vi "Dialog Window with Option.vi"(8 "Error In":errorcluster, 9 "Button 2 (Cancel)":string="Cancel", 10 "Button 1 (OK)":string="OK", 11 "Message":string) -> (0 "Error Out":errorcluster, 1 "Cancelled?":bool, 3 "OK?":bool)   [LabVIEW 2019]
panel:
  in  "Cancel":bool
  in  "OK":bool
  in  "Do not show this warning again":bool
  out "Displayed Message":string
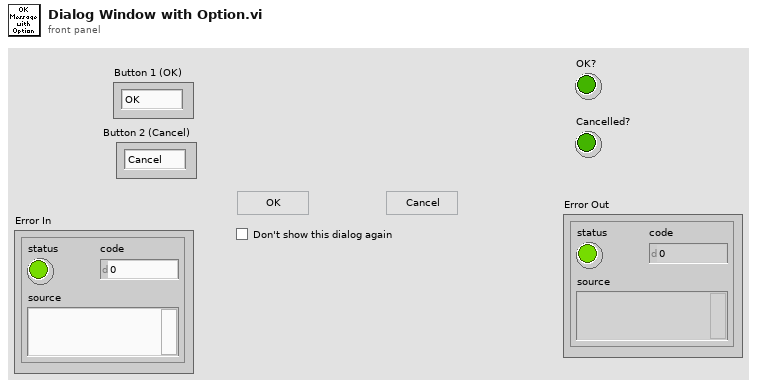
[diagram p1: front panel]
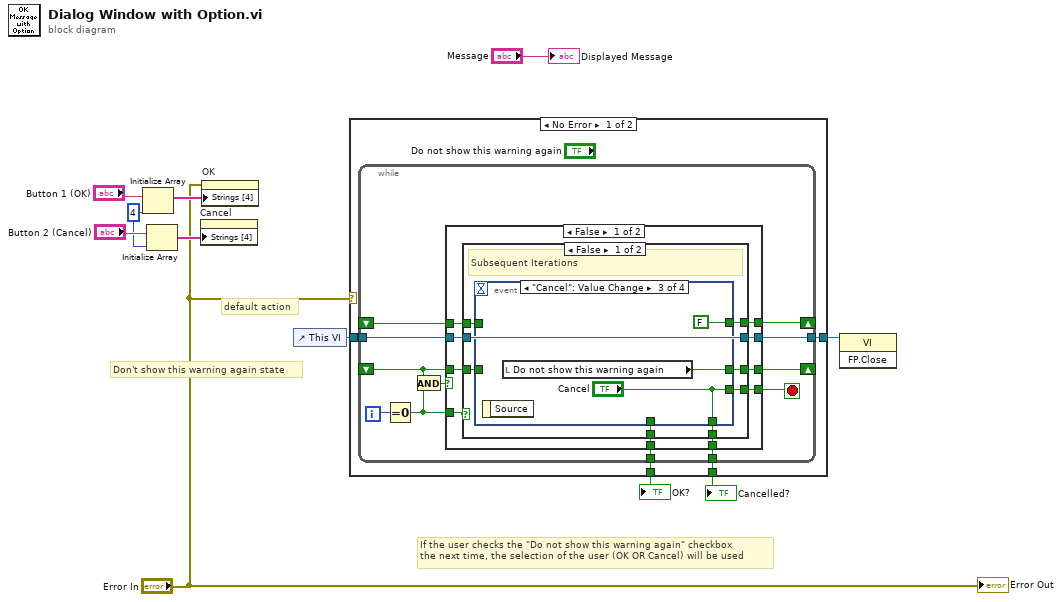
[diagram p0: block diagram]
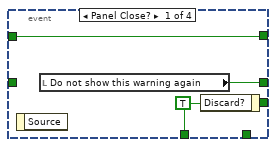
[diagram p2: hidden frame]
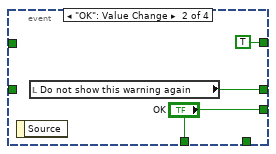
[diagram p3: hidden frame]
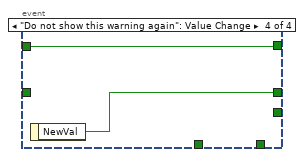
[diagram p4: hidden frame]
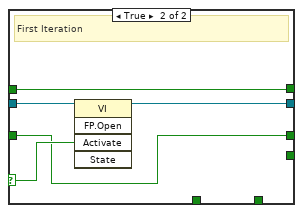
[diagram p5: hidden frame]
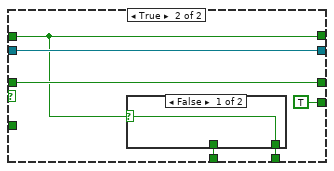
[diagram p6: hidden frame]
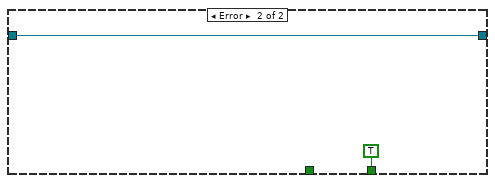
[diagram p8: hidden frame]
diagram:
  w3 = 4 ("dimension size")
  # "default action"
  # "Don't show this warning again state"
  # "If the user checks the \"Do not show this warning again\" checkbox\nthe next time, the selection of the user (OK OR Cancel) will be used"
  n1 = Initialize Array("Button 1 (OK)", w3) -> (w5:string[])
  n2 = Initialize Array("Button 2 (Cancel)", w3) -> (w2:string[])
  n3 = property on="Cancel" class="Bool"("Strings [4]"=w2) -> ()  [unwired: 2 in, 2 out]
  n4 = property on="OK" class="Bool"(error in="Error In", "Strings [4]"=w5) -> ()  [unwired: 1 in, 2 out]
  n5 = control-ref of="This VI"() -> (w10:refnum<vi>)
  n6 = case shown="No Error" "Error In" {
    tunnel: w10 -> [w15 w71]
    tunnel: [w14 w71] -> w9
    tunnel: [w13 _] -> w8
    tunnel: [w12 TRUE ("Cancel")] -> w7
    frame No Error {
      n7 = while {
        shift-right: [w27] -> _
        shift-left: _ -> [w25]
        tunnel: w15 -> [w21]
        tunnel: [w20] -> w14
        tunnel: [w19] -> w13
        tunnel: [w18] -> w12
        shift-right: [w17] -> _
        shift-left: _ -> [w16]
        i -> [w26]
        stop <- w23 stop-if-true
        n8 = Equal To 0?(x=w26) -> (x = 0?=w22:bool)
        n9 = And(x=w25, y=w22) -> (x .and. y?=w24:bool)
        n10 = case shown="False" w24 {
          tunnel: [w37 TRUE ("Cancel")] -> w23
          tunnel: [w36 w65] -> w27
          tunnel: w25 -> [w35 w65]
          tunnel: w22 -> [w34 _]
          tunnel: w21 -> [w33 w67]
          tunnel: [w32 w67] -> w20
          tunnel: [w31 w63] -> w19
          tunnel: [w30 w62] -> w18
          tunnel: [w29 w64] -> w17
          tunnel: w16 -> [w28 w64]
          frame False {
            n11 = case shown="False" w34 {
              selector: w34 -> [_ w60]
              tunnel: [w45 _] -> w37
              tunnel: [w44 w58] -> w36
              tunnel: w35 -> [w43 w58]
              tunnel: w33 -> [w42 w61]
              tunnel: [w42 w59] -> w32
              tunnel: [w41 _] -> w31
              tunnel: [w40 _] -> w30
              tunnel: [w39 w57] -> w29
              tunnel: w28 -> [w38 w57]
              frame False {
                # "Subsequent Iterations"
                n12 = event shown="[2] \"Cancel\": Value Change" {
                  selector: _ -> [_ _ _ _]
                  dyn-events: _ -> [_ _ _ _]
                  timeout: _ -> [_ _ _ _]
                  tunnel: [w47 "OK" "Cancel" _] -> w45
                  tunnel: [w48 w51 w53 w56] -> w44
                  tunnel: w43 -> [_ _ _ _]
                  tunnel: [w47 "OK" _ _] -> w41
                  tunnel: [_ _ "Cancel" _] -> w40
                  tunnel: [w46 TRUE ("Cancel") FALSE ("Cancel") w55] -> w39
                  tunnel: w38 -> [w46 _ _ w55]
                  event Panel Close? {
                    w47 = TRUE ("Discard?")
                    n13 = event-data() -> ()  [unwired: 1 in, 1 out]
                    n14 = local read "Do not show this warning again"() -> (w48:bool)
                    n15 = event-data("Discard?"=w47) -> ()  [unwired: 1 in, 1 out]
                  }
                  event "OK": Value Change {
                    n16 = event-data() -> ()  [unwired: 1 in, 1 out]
                    n17 = local read "Do not show this warning again"() -> (w51:bool)
                  }
                  event "Cancel": Value Change {
                    n18 = event-data() -> ()  [unwired: 1 in, 1 out]
                    n19 = local read "Do not show this warning again"() -> (w53:bool)
                  }
                  event "Do not show this warning again": Value Change {
                    n20 = event-data() -> ("NewVal"=w56:bool)  [unwired: 1 in]
                  }
                }
              }
              frame True {
                # "First Iteration"
                n21 = invoke class="VI" method="FP.Open"(reference=w61, "Activate"=w60) -> (reference out=w59:refnum<vi>)  [unwired: 3 in, 4 out]
              }
            }
          }
          frame True {
            n22 = case shown="False" w64 {
              selector: w64 -> [w68 w69]
              tunnel: [_ w69] -> w63
              tunnel: [w68 _] -> w62
              frame False {
              }
              frame True {
              }
            }
          }
        }
      }
    }
    frame Error {
    }
  }
  "OK?" <- w8
  "Cancelled?" <- w7
  n23 = invoke class="VI" method="FP.Close"(reference=w9) -> ()  [unwired: 2 in, 3 out]
  "Displayed Message" <- "Message"
  "Error Out" <- "Error In"
